vi "Get json value.vi"(8 "error in (no error)":errorcluster, 10 "Token prefix":string, 11 "String in":string) -> (0 "error out":errorcluster, 3 "String after prefix to endquote":string)   [LabVIEW 2013]
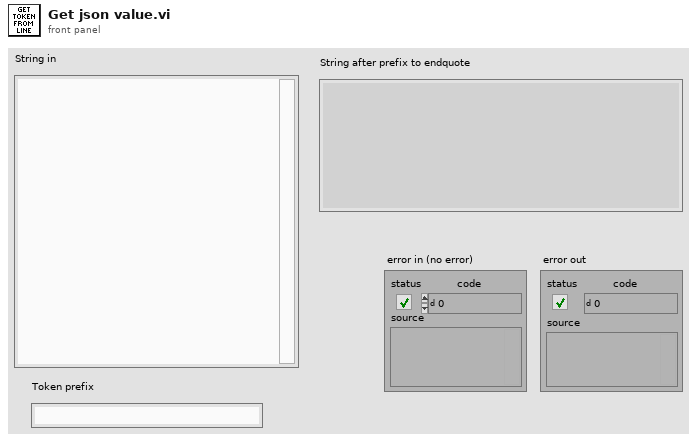
[diagram p1: front panel]
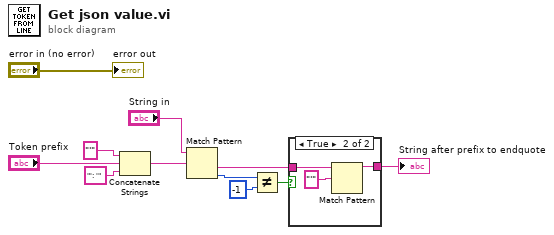
[diagram p0: block diagram]
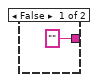
[diagram p2: hidden frame]
diagram:
  n1 = Concatenate Strings("'" ("string"), "Token prefix", "': '" ("string")) -> (w2:string)
  n2 = Match Pattern(string="String in", regular expression=w2) -> (after substring=w10:string, offset past match=w7:i32)  [unwired: 1 in, 2 out]
  n3 = Not Equal?(x=w7, y=-1) -> (x != y?=w9:bool)
  n4 = case shown="True" w9 {
    tunnel: w10 -> [_ w15]
    tunnel: ["" ("read buffer") w13] -> w11
    frame False {
    }
    frame True {
      n5 = Match Pattern(string=w15, regular expression="'") -> (before substring=w13:string)  [unwired: 1 in, 3 out]
    }
  }
  "String after prefix to endquote" <- w11
  "error out" <- "error in (no error)"
